vi "temperatureSettlingView.vi"(10 "UserEvents in":refnum<class "UserEvents.lvclass">) -> ()   [LabVIEW 2013, in "AITDTViews.lvlib"]
uses:
  AITDTViews.lvlib
  UserEvents/UserEvents.lvclass
  Typedefs/TemperatureSettling.ctl
  UserEvents/UserEvents.lvclass/UserEvents.ctl
  Typedefs/StateSelector.ctl
  Typedefs/AITDTTypedefs.lvlib
panel:
  out "TemperatureSettling":T1={"Temperature Measured"=275.15, "TemperatureSettledIsTrue"=FALSE, "Required"={"Sample Size Rqd"=0, "StDev"=275.15}, "Measured"={"StDev Msd"=275.15, "Sample Size Msd"=0}} {"Measured"."StDev Msd" min=271.15 max=275.15 format="%.4f"; "Measured"."Sample Size Msd" min=1; "Required"."Sample Size Rqd" min=1; "Required"."StDev" min=271.15 max=275.15 format="%.4f"; "Temperature Measured" min=271.15 max=275.15 format="%.1f"}
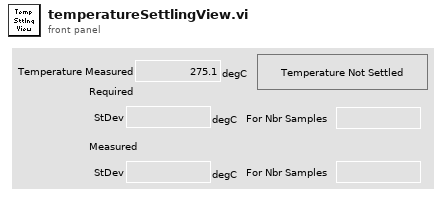
[diagram p1: front panel]
types:
  T1 = typedef "AITDTTypedefs.lvlib/TemperatureSettling.ctl" = cluster{"Temperature Measured":dbl[unit], "TemperatureSettledIsTrue":bool, "Required":cluster{"Sample Size Rqd":u16, "StDev":dbl[unit]}, "Measured":cluster{"StDev Msd":dbl[unit], "Sample Size Msd":u16}}
  T2 = typedef "AITDTTypedefs.lvlib/PubDataEvents.ctl" = cluster{"State":refnum<user-event>, "ErrorCode":refnum<user-event>, "OutputData":refnum<user-event>, "InputData":refnum<user-event>, "TestStatus":refnum<user-event>, "LogPath":refnum<user-event>, "TemperatureSetpointRequest":refnum<user-event>, "TemperatureSettling":refnum<user-event>, "WaitTimeStatus":refnum<user-event>}
  T3 = cluster{"Event Registration Refnum":refnum<event-registration>, "Event Registration Refnum":refnum<event-registration>}
  T4 = typedef "AITDTTypedefs.lvlib/StateSelector.ctl" = enum16{"AwaitingSetpointAcknowledgmentState", "EndingCycleState", "FaultState", "OffState", "PausingState", "RequestingNewSetpointState", "SamplingState", "SettlingState", "SoakingState", "StabilizingState", "StandbyState", "StoppedState", "TransitioningTemperatureState"}
  T5 = cluster{"Sample Size Rqd":u16, "StDev":dbl[unit]}
  T6 = cluster{"StDev Msd":dbl[unit], "Sample Size Msd":u16}
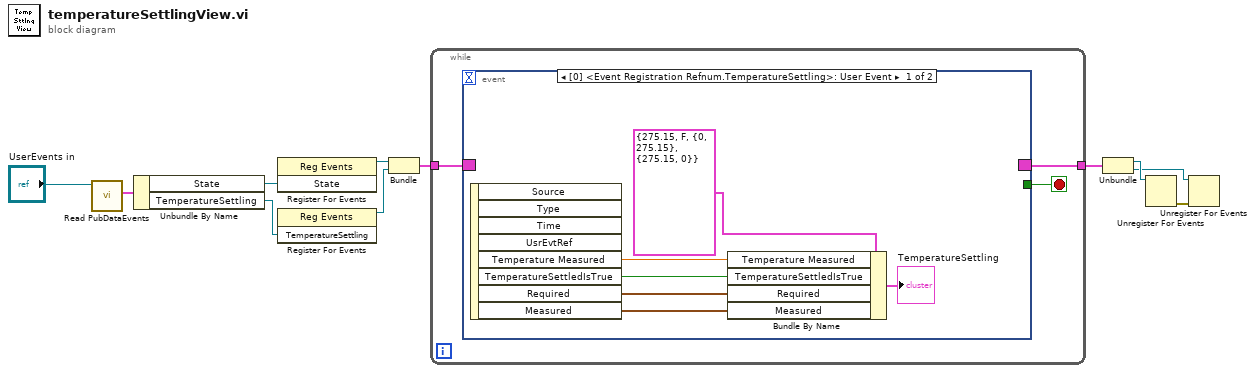
[diagram p0: block diagram]
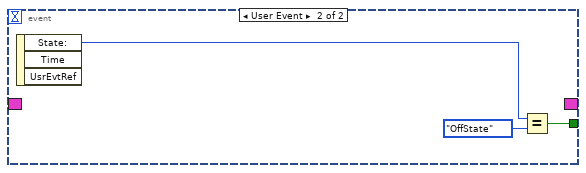
[diagram p2: hidden frame]
diagram:
  n1 = call "Read PubDataEvents.vi"("UserEvents in"="UserEvents in") -> ("PubDataEvents"=w11:T2)  [unwired: 9 in, 1 out]
  n2 = Unbundle By Name(w11) -> ("State"=w10:refnum<user-event>, "TemperatureSettling"=w8:refnum<user-event>)
  n3 = register-events(w10) -> (reference out=w9:refnum<event-registration>)  [unwired: 2 in, 1 out]
  n4 = register-events(w8) -> (reference out=w7:refnum<event-registration>)  [unwired: 2 in, 1 out]
  n5 = Bundle("Event Registration Refnum"=w9, "Event Registration Refnum"=w7) -> (w5:T3)  [unwired: 1 in]
  n6 = while {
    tunnel: w5 -> [w14]
    tunnel: [w12] -> w4
    stop <- w13 stop-if-true
    n7 = event shown="[0] <Event Registration Refnum.TemperatureSettling>: User Event" {
      selector: w14 -> [_ _]
      dyn-events: [_ _] -> w12
      timeout: _ -> [_ _]
      tunnel: [_ w22] -> w13
      event User Event {
        n8 = event-data() -> ("Temperature Measured"=w19:dbl[unit], "TemperatureSettledIsTrue"=w18:bool, "Required"=w17:T5, "Measured"=w16:T6)  [unwired: 1 in, 4 out]
        n9 = Bundle By Name(cluster=T1 {"Temperature Measured"=275.15, "TemperatureSettledIsTrue"=FALSE, "Required"={"Sample Size Rqd"=0, "StDev"=275.15}, "Measured"={"StDev Msd"=275.15, "Sample Size Msd"=0}} ("TemperatureSettling"), "Temperature Measured"=w19, "TemperatureSettledIsTrue"=w18, "Required"=w17, "Measured"=w16) -> (→"TemperatureSettling":T1)
      }
      event User Event {
        n10 = event-data() -> ("State:"=w21:T4)  [unwired: 1 in, 2 out]
        n11 = Equal?(x=w21, y=StateSelector."OffState" ("State:")) -> (x = y?=w22:bool)
      }
    }
  }
  n12 = Unbundle(w4) -> ("Event Registration Refnum"=w3:refnum<event-registration>, "Event Registration Refnum"=w2:refnum<event-registration>)
  n13 = Unregister For Events(event registration refnum=w3) -> (error out=w1:errorcluster)  [unwired: 1 in]
  n14 = Unregister For Events(event registration refnum=w2, error in=w1) -> ()  [unwired: 1 out]
